vi "Save As Bmp.vi"(7 "ymax":i32, 8 "error in (no error)":errorcluster, 9 "ymin":i32, 10 "palette":string, 11 "path":string) -> (0 "error out":errorcluster, 3 "function return":u32)   [LabVIEW 2014, in "atmcd32d.lvlib"]
doc: "unsigned int WINAPI SaveAsBmp(const char * path, const char * palette, long ymin, long ymax);"
uses:
  atmcd32d.lvlib
  atmcd32d.dll
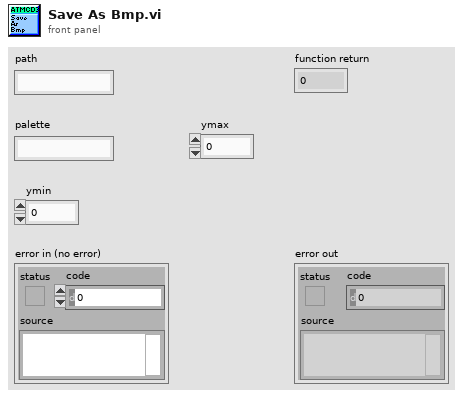
[diagram p1: front panel]
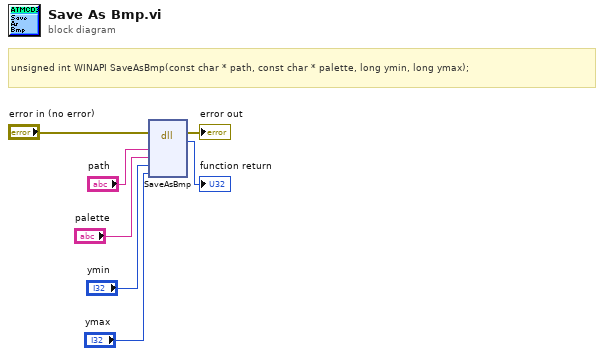
[diagram p0: block diagram]
diagram:
  # "unsigned int WINAPI SaveAsBmp(const char * path, const char * palette, long ymin, long ymax);"
  n1 = dll-call lib="C:/Users/Bakir/Documents/Lambda2-Testing/lib/Andorlib/atmcd32d.*" fn="SaveAsBmp"(error in="error in (no error)", "path"="path", "palette"="palette", "ymin"="ymin", "ymax"="ymax") -> (error out=→"error out":errorcluster, →"function return":u32)  [unwired: 6 in, 1 out]
